vi "Read RIO interface.vi"(8 "error in":errorcluster, 11 "Profibus Module configuration in":refnum<class "Profibus Module configuration.lvclass">) -> (0 "error out":errorcluster, 2 "RIO interface":string="RIO0", 3 "Profibus Module configuration out":refnum<class "Profibus Module configuration.lvclass">)   [LabVIEW 2013, in "Profibus Module configuration.lvclass"]
uses:
  Profibus Module configuration.lvclass
  Profibus Module configuration.lvclass/Profibus Module configuration.ctl
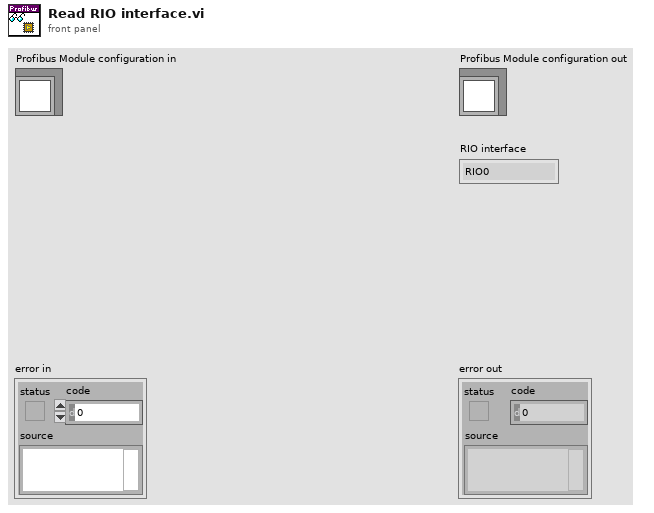
[diagram p1: front panel]
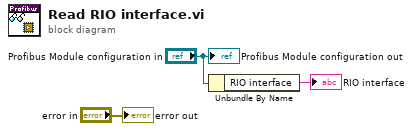
[diagram p0: block diagram]
diagram:
  n1 = Unbundle By Name("Profibus Module configuration in") -> ("RIO interface"=→"RIO interface":string)
  "error out" <- "error in"
  "Profibus Module configuration out" <- "Profibus Module configuration in"
